vi "Standby.vi"(8 "error in (no error)":errorcluster, 10 "Model in":refnum<class "Model.lvclass">, 11 "Disabled State in":refnum<class "Disabled State.lvclass">) -> (0 "error out":errorcluster, 2 "Model out":refnum<class "Model.lvclass">, 3 "Disabled State out":refnum<class "Disabled State.lvclass">)   [LabVIEW 2015, in "Disabled State.lvclass"]
uses:
  Disabled State.lvclass
  Model/Model/Model.lvclass
  Typedefs/State Types.ctl
  Typedefs/FAMT Typedefs.lvlib
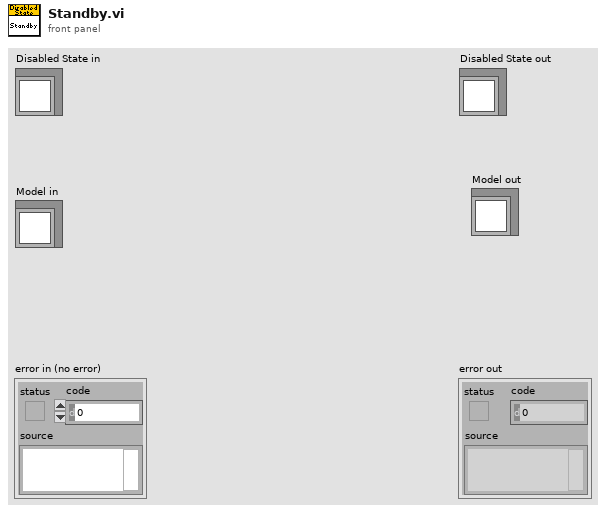
[diagram p1: front panel]
types:
  T1 = typedef "FAMT Typedefs.lvlib/State Types.ctl" = enum16{"Offline State", "Fault State", "Standby State", "Disabled State", "Enabled State", "Wait For User Input State", "Perform Open Loop Scan State", "Perform Closed Loop Scan State"}
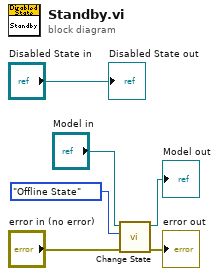
[diagram p0: block diagram]
diagram:
  n1 = call "Change State.vi"("error in (no error)"="error in (no error)", "State Types"=State_Types."Offline State" ("State:"), "Model in"="Model in") -> ("error out"=→"error out":errorcluster, "Model out"=→"Model out":refnum<class "Model.lvclass">)  [unwired: 7 in]
  "Disabled State out" <- "Disabled State in"
